vi "ERIO WIN Update Supervisory Variables.vi"(6 "Supervisory Variables In":T3={"Alarm Threshold"=0.0, "Shutdown"=FALSE, "Enable SNS Alarm"=FALSE, "Enable SNS Stage Notification"=FALSE, "Enable SQS Notification"=FALSE, "Enable S3 TDMS Signal Capture"=FALSE, "Enable SystemLink Signal Capture"=FALSE, "Capture Signal"=FALSE, "Server Update"=FALSE, "AWS Access Key"="AKIAINLDO2Y2PDFEWDOQ", "AWS Secret Key"="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", "Phone Number"="+15037066913", "Region"=enum."us-west-2", "AWS SQS Queue"="+15037066913", "AWS S3 Bucket"="+15037066913"}, 7 "WIN State In":T1, 8 "error in (no error)":errorcluster, 9 "AWS Variables In":T5, 11 "EEISysLink.lvclass In":refnum<class "EEISysLink.lvclass">) -> (0 "error out":errorcluster, 1 "AWS Variables Out":T5, 3 "EEISysLink.lvclass Out":refnum<class "EEISysLink.lvclass">, 4 "Supervisory Variables Out":T3={"Alarm Threshold"=0.0, "Shutdown"=FALSE, "Enable SNS Alarm"=FALSE, "Enable SNS Stage Notification"=FALSE, "Enable SQS Notification"=FALSE, "Enable S3 TDMS Signal Capture"=FALSE, "Enable SystemLink Signal Capture"=FALSE, "Capture Signal"=FALSE, "Server Update"=FALSE, "AWS Access Key"="AKIAINLDO2Y2PDFEWDOQ", "AWS Secret Key"="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", "Phone Number"="+15037066913", "Region"=enum."us-west-2", "AWS SQS Queue"="+15037066913", "AWS S3 Bucket"="+15037066913"}, 5 "WIN State Out":T1)   [LabVIEW 2017]
doc: "Use worker, notifier, signal, and UI information to process for supervisory variable update as indicated. \n\nJames Tillett P.E.\nEndeavor Engineering Inc.\nwww.endeavoreng.com"
uses:
  Class EEISysLink/EEISysLink.lvclass
  Controls/ERIO AWS Toolkit Variables.ctl
  <vilib>/AWS Toolkit/SQS/Queue/Queue.lvclass
  <vilib>/AWS Toolkit/SNS/Phone Number/Phone Number.lvclass
  <vilib>/AWS Toolkit/S3/Bucket/Bucket.lvclass
  Controls/ERIO Supervisory Variables.ctl
  <vilib>/AWS Toolkit/Core/HTTP Request/Region.ctl
  Controls/ERIO WIN State Variables.ctl
  Controls/ERIO Worker Variables.ctl
  Class EEISysLink/Controls/SL Tag Type.ctl
  Class EEISysLink/Controls/SL Tag Data Type.ctl
  Class EEISysLink/Controls/SL Tag Scope.ctl
  Class EEISysLink/Controls/SL Tag Value.ctl
  <vilib>/AWS Toolkit/Core/HTTP Request/HTTP Request.lvclass
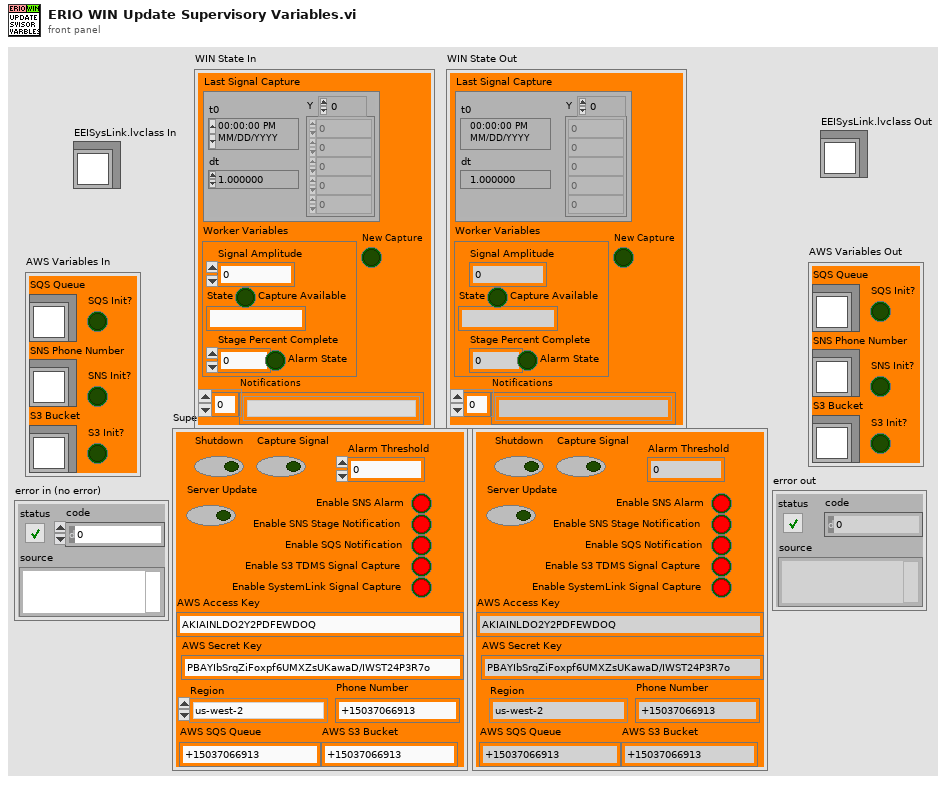
[diagram p1: front panel]
types:
  T1 = typedef "ERIO WIN State Variables.ctl" = cluster{"Worker Variables":T2, "Notifications":string[], "New Capture":bool, "Last Signal Capture":waveform(dbl)}
  T2 = typedef "ERIO Worker Variables.ctl" = cluster{"Signal Amplitude":dbl, "State":string, "Stage Percent Complete":dbl, "Alarm State":bool, "Capture Available":bool}
  T3 = typedef "ERIO Supervisory Variables.ctl" = cluster{"Alarm Threshold":dbl, "Shutdown":bool, "Enable SNS Alarm":bool, "Enable SNS Stage Notification":bool, "Enable SQS Notification":bool, "Enable S3 TDMS Signal Capture":bool, "Enable SystemLink Signal Capture":bool, "Capture Signal":bool, "Server Update":bool, "AWS Access Key":string, "AWS Secret Key":string, "Phone Number":string, "Region":T4, "AWS SQS Queue":string, "AWS S3 Bucket":string}
  T4 = typedef "NI_AWS_Core.lvlib/HTTP Request.lvclass/Region.ctl" = enum16{"us-east-1", "us-east-2", "us-west-1", "us-west-2", "ap-northeast-1", "ap-northeast-2", "ap-southeast-1", "ap-southeast-2", "ca-central-1", "eu-central-1", "eu-west-1", "eu-west-2", "sa-east-1"}
  T5 = typedef "ERIO AWS Toolkit Variables.ctl" = cluster{"SQS Queue":refnum<class "Queue.lvclass">, "SNS Phone Number":refnum<class "Phone Number.lvclass">, "S3 Bucket":refnum<class "Bucket.lvclass">, "SQS Init?":bool, "S3 Init?":bool, "SNS Init?":bool}
  T6 = typedef "EEISysLink.lvclass/SL Tag Data Type.ctl" = enum16{"Double", "Integer", "String", "Boolean", "Waveform"}
  T7 = typedef "EEISysLink.lvclass/SL Tag Scope.ctl" = enum16{"Local", "Server"}
  T8 = typedef "EEISysLink.lvclass/SL Tag Type.ctl" = enum16{"All", "Supervisor", "Worker"}
  T9 = typedef "SL Tag Value.ctl" = cluster{"Value":variant, "Time Stamp":timestamp, "Tag Data Type":T6, "Name":string}
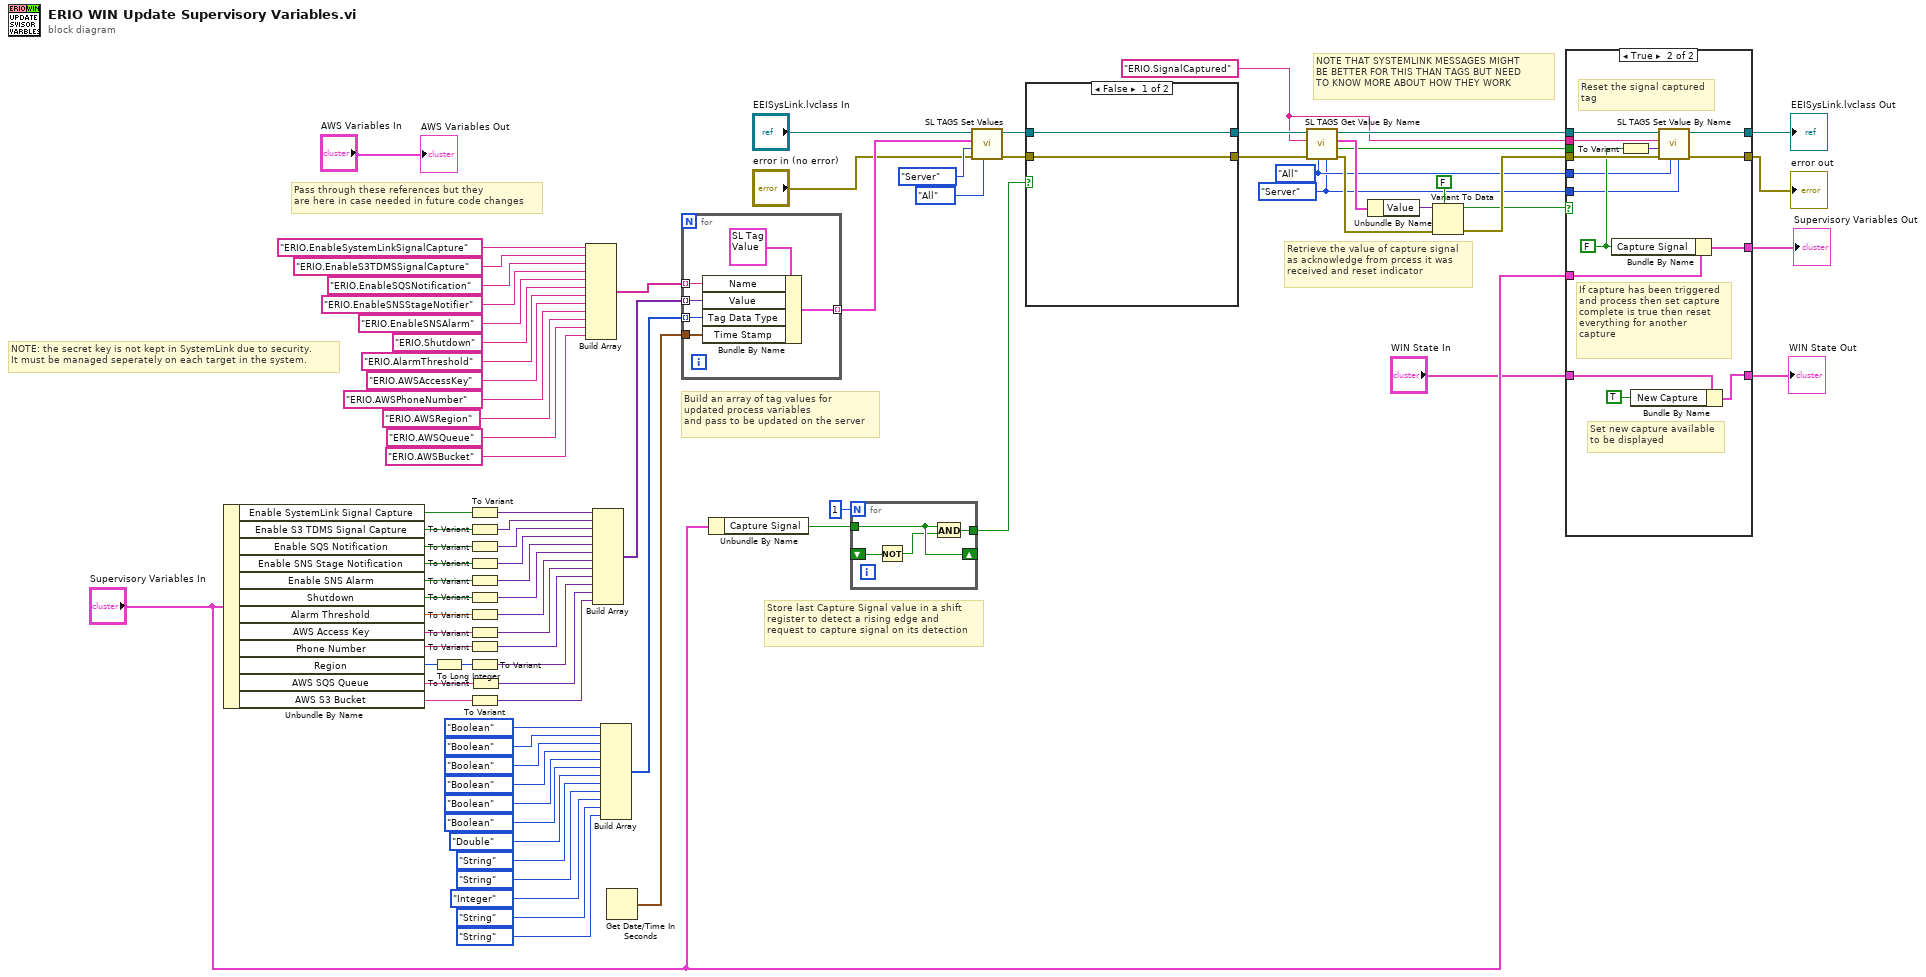
[diagram p0: block diagram]
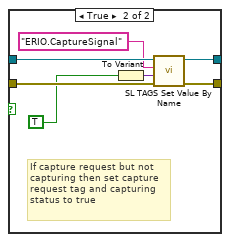
[diagram p3: hidden frame]
diagram:
  w33 = "ERIO.SignalCaptured"
  w28 = SL_Tag_Scope."Server" ("Tag Scope")
  w29 = SL_Tag_Type."All" ("Tag Type")
  # "NOTE: the secret key is not kept in SystemLink due to security.\nIt must be managed seperately on each target in the system."
  # "Store last Capture Signal value in a shift\nregister to detect a rising edge and\nrequest to capture signal on its detection"
  # "NOTE THAT SYSTEMLINK MESSAGES MIGHT\nBE BETTER FOR THIS THAN TAGS BUT NEED \nTO KNOW MORE ABOUT HOW THEY WORK"
  # "Retrieve the value of capture signal\nas acknowledge from prcess it was\nreceived and reset indicator"
  # "Build an array of tag values for\nupdated process variables\nand pass to be updated on the server"
  # "Pass through these references but they\nare here in case needed in future code changes"
  n1 = Unbundle By Name("Supervisory Variables In") -> ("Enable SystemLink Signal Capture"=w82:bool, "Enable S3 TDMS Signal Capture"=w81:bool, "Enable SQS Notification"=w80:bool, "Enable SNS Stage Notification"=w79:bool, "Enable SNS Alarm"=w78:bool, "Shutdown"=w77:bool, "Alarm Threshold"=w76:dbl, "AWS Access Key"=w14:string, "Phone Number"=w15:string, "Region"=w16:T4, "AWS SQS Queue"=w2:string, "AWS S3 Bucket"=w1:string)
  n2 = To Long Integer(number=w16) -> (32bit integer=w17:i32)
  n3 = To Variant(anything=w82) -> (Variant=w68:variant)
  n4 = To Variant(anything=w81) -> (Variant=w67:variant)
  n5 = To Variant(anything=w80) -> (Variant=w66:variant)
  n6 = To Variant(anything=w79) -> (Variant=w65:variant)
  n7 = To Variant(anything=w78) -> (Variant=w64:variant)
  n8 = To Variant(anything=w77) -> (Variant=w63:variant)
  n9 = To Variant(anything=w76) -> (Variant=w62:variant)
  n10 = To Variant(anything=w14) -> (Variant=w13:variant)
  n11 = To Variant(anything=w15) -> (Variant=w12:variant)
  n12 = To Variant(anything=w17) -> (Variant=w11:variant)
  n13 = To Variant(anything=w1) -> (Variant=w3:variant)
  n14 = To Variant(anything=w2) -> (Variant=w4:variant)
  n15 = Build Array("ERIO.EnableSystemLinkSignalCapture", "ERIO.EnableS3TDMSSignalCapture", "ERIO.EnableSQSNotification", "ERIO.EnableSNSStageNotifier", "ERIO.EnableSNSAlarm", "ERIO.Shutdown", "ERIO.AlarmThreshold", "ERIO.AWSAccessKey", "ERIO.AWSPhoneNumber", "ERIO.AWSRegion", "ERIO.AWSQueue", "ERIO.AWSBucket") -> (w52:string[])
  n16 = Build Array(w68, w67, w66, w65, w64, w63, w62, w13, w12, w11, w4, w3) -> (w51:variant[])
  n17 = Build Array(SL_Tag_Data_Type."Boolean" ("Tag Data Type"), SL_Tag_Data_Type."Boolean" ("Tag Data Type"), SL_Tag_Data_Type."Boolean" ("Tag Data Type"), SL_Tag_Data_Type."Boolean" ("Tag Data Type"), SL_Tag_Data_Type."Boolean" ("Tag Data Type"), SL_Tag_Data_Type."Boolean" ("Tag Data Type"), SL_Tag_Data_Type."Double" ("Tag Data Type"), SL_Tag_Data_Type."String" ("Tag Data Type"), SL_Tag_Data_Type."String" ("Tag Data Type"), SL_Tag_Data_Type."Integer" ("Tag Data Type"), SL_Tag_Data_Type."String" ("Tag Data Type"), SL_Tag_Data_Type."String" ("Tag Data Type")) -> (w50:T6[])
  n18 = Get Date/Time In Seconds() -> (seconds since 1Jan1904=w49:timestamp)
  n19 = for {
    tunnel: w52 -> [w88] mode=indexing
    tunnel: w51 -> [w87] mode=indexing
    tunnel: w50 -> [w86] mode=indexing
    tunnel: w49 -> [w85]
    tunnel: [w84] -> w48 mode=indexing
    n20 = Bundle By Name(cluster=T9 {"Value"=variant, "Time Stamp"=timestamp(0 s since 1904-01-01), "Tag Data Type"=enum."Double", "Name"=""} ("Tag Value"), "Name"=w88, "Value"=w87, "Tag Data Type"=w86, "Time Stamp"=w85) -> (w84:T9)
  }
  n21 = Unbundle By Name("Supervisory Variables In") -> ("Capture Signal"=w26:bool)
  n22 = for {
    N: 1 -> [_]
    tunnel: [w93] -> w41
    tunnel: w26 -> [w92]
    shift-right: [w92] -> _
    shift-left: _ -> [w91]
    n23 = Not(x=w91) -> (.not. x?=w90:bool)
    n24 = And(x=w92, y=w90) -> (x .and. y?=w93:bool)
  }
  n25 = call-dynamic "SL TAGS Set Values.vi"("Tag Type"=SL_Tag_Type."All", "error in (no error)"="error in (no error)", "Tag Scope"=SL_Tag_Scope."Server", "Tag Update Values"=w48, "EEISysLink in"="EEISysLink.lvclass In") -> ("error out"=w39:errorcluster, "EEISysLink out"=w40:refnum<class "EEISysLink.lvclass">)  [unwired: 5 in]
  n26 = case shown="False" w41 {
    tunnel: w40 -> [w95 w102]
    tunnel: [w95 w101] -> w38
    tunnel: w39 -> [w94 w99]
    tunnel: [w94 w98] -> w37
    frame False {
    }
    frame True {
      # "If capture request but not\ncapturing then set capture\nrequest tag and capturing\nstatus to true"
      n27 = To Variant(anything=TRUE ("Capturing Signal")) -> (Variant=w100:variant)
      n28 = call-dynamic "SL TAGS Set Value By Name.vi"("error in (no error)"=w99, "Value"=w100, "Tag Name"="ERIO.CaptureSignal", "EEISysLink in"=w102) -> ("error out"=w98:errorcluster, "EEISysLink out"=w101:refnum<class "EEISysLink.lvclass">)  [unwired: 6 in]
    }
  }
  n29 = call-dynamic "SL TAGS Get Value By Name.vi"("Tag Scope"=w28, "Tag Type"=w29, "error in (no error)"=w37, "Tag Name"=w33, "EEISysLink in"=w38) -> ("error out"=w42:errorcluster, "Found?"=w30:bool, "Tag Value"=w45:T9, "EEISysLink out"=w35:refnum<class "EEISysLink.lvclass">)  [unwired: 3 in]
  n30 = Unbundle By Name(w45) -> ("Value"=w44:variant)
  n31 = Variant To Data(error in=w42, type=FALSE, Variant=w44) -> (data=w27:bool, error out=w34:errorcluster)
  n32 = case shown="True" w27 {
    tunnel: "Supervisory Variables In" -> [w104 w120]
    tunnel: [w104 w119] -> w36
    tunnel: w35 -> [w106 w117]
    tunnel: w34 -> [w105 w116]
    tunnel: w33 -> [_ w115]
    tunnel: [w105 w113] -> w32
    tunnel: [w106 w112] -> w31
    tunnel: w30 -> [_ _]
    tunnel: w29 -> [_ w111]
    tunnel: w28 -> [_ w110]
    tunnel: "WIN State In" -> [w103 w109]
    tunnel: [w103 w107] -> w9
    frame False {
      # "Signal capture not \nacknowledged"
    }
    frame True {
      w114 = FALSE ("Capture Signal")
      # "Set new capture available\nto be displayed"
      # "Reset the signal captured\ntag"
      # "If capture has been triggered\nand process then set capture\ncomplete is true then reset\neverything for another\ncapture"
      n33 = Bundle By Name(cluster=w120, "Capture Signal"=w114) -> (w119:T3)
      n34 = To Variant(anything=w114) -> (Variant=w118:variant)
      n35 = Bundle By Name(cluster=w109, "New Capture"=TRUE) -> (w107:T1)
      n36 = call-dynamic "SL TAGS Set Value By Name.vi"("Tag Scope"=w110, "Tag Type"=w111, "error in (no error)"=w116, "Value"=w118, "Tag Name"=w115, "EEISysLink in"=w117) -> ("error out"=w113:errorcluster, "EEISysLink out"=w112:refnum<class "EEISysLink.lvclass">)  [unwired: 4 in]
    }
  }
  "error out" <- w32
  "EEISysLink.lvclass Out" <- w31
  "Supervisory Variables Out" <- w36
  "WIN State Out" <- w9
  "AWS Variables Out" <- "AWS Variables In"
